vi "Close File Do.vi"(8 "error in (no error)":errorcluster, 10 "File Path":path, 11 "File Writer in":refnum<class "File Writer.lvclass">) -> (0 "error out":errorcluster, 3 "File Writer out":refnum<class "File Writer.lvclass">)   [LabVIEW 2020, in "File Writer.lvlib" / "File Writer.lvclass"]
doc: "Close file."
uses:
  File Writer.lvclass
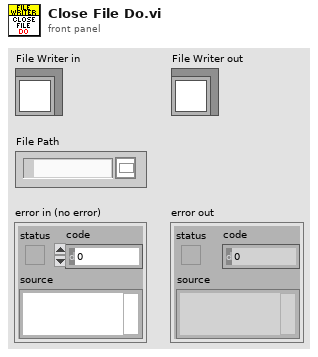
[diagram p1: front panel]
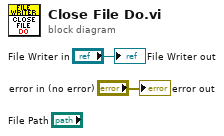
[diagram p0: block diagram]
diagram:
  "error out" <- "error in (no error)"
  "File Writer out" <- "File Writer in"
